vi "Unflatten.vi"(8 "error in (no error)":errorcluster, 11 "multimeter reader in":refnum<class "multimeter reader.lvclass">) -> (0 "error out":errorcluster, 3 "multimeter reader out":refnum<class "multimeter reader.lvclass">)   [LabVIEW 2012, in "multimeter reader.lvclass"]
uses:
  multimeter reader.lvclass
  Reader/Reader.lvclass
  multimeter reader.lvclass/multimeter reader.ctl
  Global/File Locations.vi
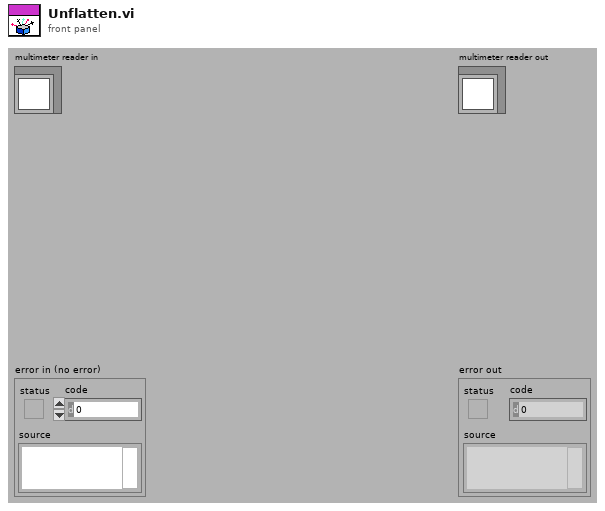
[diagram p1: front panel]
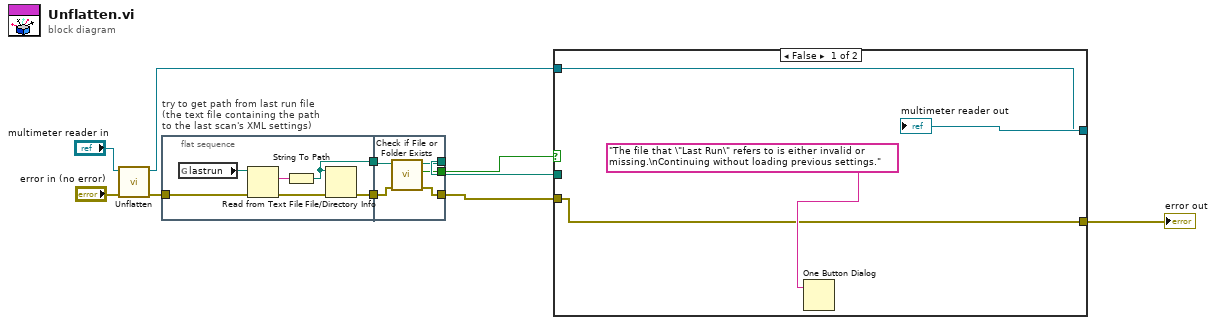
[diagram p0: block diagram]
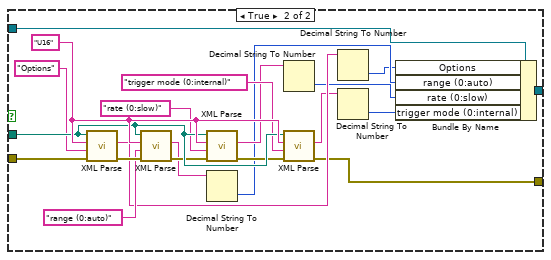
[diagram p2: hidden frame]
diagram:
  n1 = call-parent "Unflatten.vi"("error in (no error)"="error in (no error)", "Reader in"="multimeter reader in") -> ("error out"=w8:errorcluster, "Reader out"=w11:refnum<class "multimeter reader.lvclass">)  [unwired: 8 in]
  n2 = flat-sequence "try to get path from last run file\n(the text file containing the path\nto the last scan's XML settings)" {
    tunnel: w8 -> [w12]
    tunnel: [w17] -> w3
    tunnel: [w13] -> w2
    tunnel: [w21] -> w5
    tunnel: [w22] -> w6
    tunnel: w3 -> [w19]
    tunnel: w2 -> [w20]
    tunnel: [w18] -> w1
    frame #0 {
      n3 = global read "File Locations.vi" "lastrun"() -> (w15:path)
      n4 = Read from Text File(file (use dialog)=w15, error in=w12) -> (text=w16:string, error out=w14:errorcluster)  [unwired: 4 out]
      n5 = String To Path(string=w16) -> (path=w17:path)
      n6 = File/Directory Info(path=w17, error in=w14) -> (error out=w13:errorcluster)  [unwired: 6 out]
    }
    frame #1 {
      n7 = call <vilib>:"Check if File or Folder Exists.vi"("error in (no error)"=w20, "path"=w19) -> ("error out"=w21:errorcluster, "file or folder exists?"=w18:bool, "dup path"=w22:path)  [unwired: 7 in]
    }
  }
  n8 = case shown="False" w1 {
    tunnel: w11 -> [w24 w46]
    tunnel: [w24 w45] -> w7
    tunnel: w6 -> [_ w43]
    tunnel: w5 -> [w23 w42]
    tunnel: [w23 w26] -> w4
    frame False {
      n9 = One Button Dialog(message="The file that \"Last Run\" refers to is either invalid or missing.\nContinuing without loading previous settings.") -> ()  [unwired: 1 in, 1 out]
    }
    frame True {
      w44 = "U16"
      n10 = call "XML Parse.vi"("error in (no error)"=w42, "Name String"="Options", "Type String"=w44, "Path"=w43) -> ("error out"=w41:errorcluster, "String Out"=w34:string)  [unwired: 6 in]
      n11 = call "XML Parse.vi"("error in (no error)"=w41, "Name String"="range (0:auto)", "Type String"=w44, "Path"=w43) -> ("error out"=w40:errorcluster, "String Out"=w33:string)  [unwired: 6 in]
      n12 = call "XML Parse.vi"("error in (no error)"=w40, "Name String"="rate (0:slow)", "Type String"=w44, "Path"=w43) -> ("error out"=w39:errorcluster, "String Out"=w32:string)  [unwired: 6 in]
      n13 = Decimal String To Number(string=w33) -> (number=w28:i32)  [unwired: 2 in, 1 out]
      n14 = Decimal String To Number(string=w32) -> (number=w29:i32)  [unwired: 2 in, 1 out]
      n15 = call "XML Parse.vi"("error in (no error)"=w39, "Name String"="trigger mode (0:internal)", "Type String"=w44, "Path"=w43) -> ("error out"=w26:errorcluster, "String Out"=w31:string)  [unwired: 6 in]
      n16 = Decimal String To Number(string=w34) -> (number=w27:i32)  [unwired: 2 in, 1 out]
      n17 = Decimal String To Number(string=w31) -> (number=w30:i32)  [unwired: 2 in, 1 out]
      n18 = Bundle By Name(cluster=w46, "Options"=w27, "range (0:auto)"=w28, "rate (0:slow)"=w29, "trigger mode (0:internal)"=w30) -> (w45:refnum<class "multimeter reader.lvclass">)
    }
  }
  "multimeter reader out" <- w7
  "error out" <- w4
